vi "invert color.vi"(10 "color":u8) -> (2 "invert color":u8)   [LabVIEW 2019, in "Userlib.lvlib"]
uses:
  Userlib.lvlib
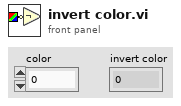
[diagram p1: front panel]
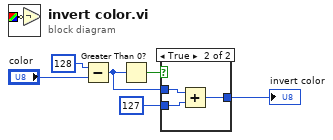
[diagram p0: block diagram]
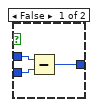
[diagram p2: hidden frame]
diagram:
  n1 = Subtract(x=u8 128 ("y"), y="color") -> (x-y=w1:u8)
  n2 = Greater Than 0?(x=w1) -> (x > 0?=w2:bool)
  n3 = case shown="True" w2 {
    tunnel: w1 -> [w9 w12]
    tunnel: u8 127 -> [w8 w11]
    tunnel: [w7 w10] -> w6
    frame False {
      n4 = Subtract(x=w9, y=w8) -> (x-y=w7:u8)
    }
    frame True {
      n5 = Add(x=w12, y=w11) -> (x+y=w10:u8)
    }
  }
  "invert color" <- w6
